vi "tt20panel_register_events.vi"(8 "error in (no error)":errorcluster, 11 "tt20panel in":refnum<class "tt20panel.lvclass">) -> (0 "error out":errorcluster, 2 "event_refs":T1, 3 "tt20panel out":refnum<class "tt20panel.lvclass">)   [LabVIEW 2015, in "tt20panel.lvclass"]
uses:
  tt20panel.lvclass
  tt20_evebnt_refs_tdef.ctl
  tt20_class/tt20_hardware_info_tdef.ctl
  tt20_acq_mode_tdef.ctl
  tt20_event_tdef.ctl
  tt20panel.lvclass/tt20panel.ctl
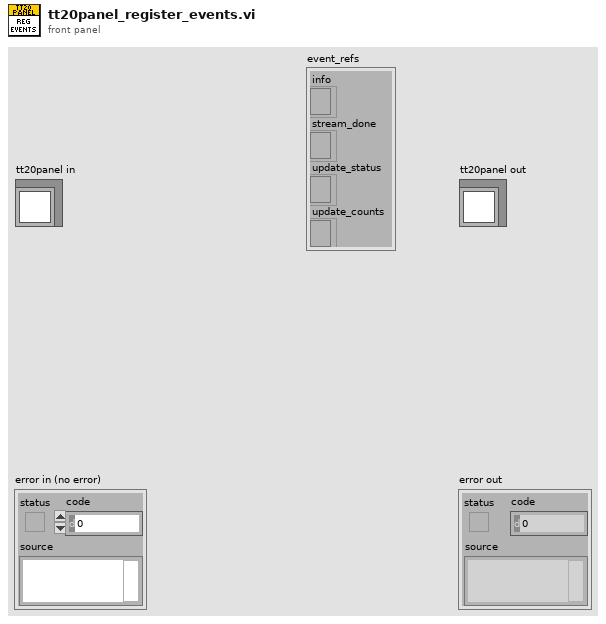
[diagram p1: front panel]
types:
  T1 = typedef "tt20_evebnt_refs_tdef.ctl" = cluster{"info":refnum<event-registration>, "stream_done":refnum<event-registration>, "update_status":refnum<event-registration>, "update_counts":refnum<event-registration>}
  T2 = typedef "tt20_event_tdef.ctl" = cluster{"tt20_get_info":refnum<user-event>, "stream_done":refnum<user-event>, "update_status":refnum<user-event>, "update_counts":refnum<user-event>}
  T3 = typedef "tt20_hardware_info_tdef.ctl" = cluster{"model":string, "serial":string, "trigger_level":dbl[], "input_delay":i64[], "deadtime":i64[], "num_channels":u32, "status":string, "enabled":bool[], "Mode":T4, "Reference Channel":u8}
  T4 = typedef "tt20_acq_mode_tdef.ctl" = enum16{"T2", "T3"}
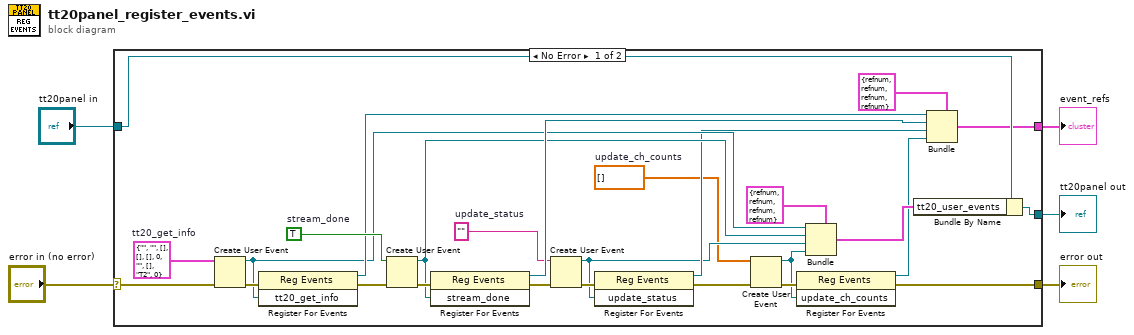
[diagram p0: block diagram]
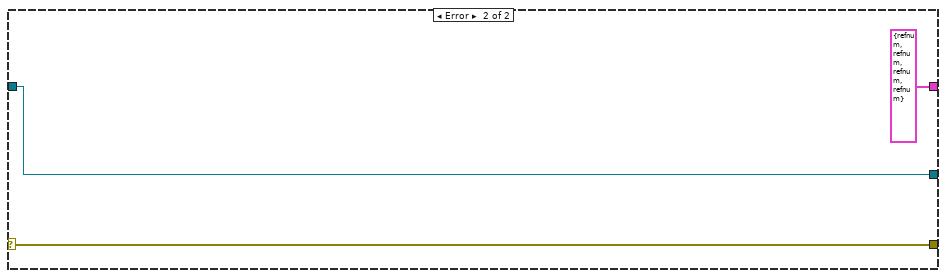
[diagram p2: hidden frame]
diagram:
  n1 = case shown="No Error" "error in (no error)" {
    selector: "error in (no error)" -> [w30 w35]
    tunnel: [w8 w35] -> w4
    tunnel: [w18 w34] -> w2
    tunnel: "tt20panel in" -> [w19 w34]
    tunnel: [w17 T1 {"info"=refnum, "stream_done"=refnum, "update_status"=refnum, "update_counts"=refnum} ("output cluster")] -> w1
    frame No Error {
      w10 = dbl[] []  # update_ch_counts
      w15 = ""  # update_status
      w31 = TRUE  # stream_done
      w32 = T3 {"model"="", "serial"="", "trigger_level"=[], "input_delay"=[], "deadtime"=[], "num_channels"=0, "status"="", "enabled"=[], "Mode"=enum."T2", "Reference Channel"=0}  # tt20_get_info
      n2 = Create User Event(user event datatype=w32, error in=w30) -> (user event=w23:refnum<user-event>, error out=w29:errorcluster)
      n3 = register-events(error in=w29, w23) -> (reference out=w25:refnum<event-registration>, error out=w28:errorcluster)  [unwired: 1 in]
      n4 = Create User Event(user event datatype=w31, error in=w28) -> (user event=w22:refnum<user-event>, error out=w27:errorcluster)
      n5 = register-events(error in=w27, w22) -> (reference out=w26:refnum<event-registration>, error out=w16:errorcluster)  [unwired: 1 in]
      n6 = Create User Event(user event datatype=w15, error in=w16) -> (user event=w12:refnum<user-event>, error out=w14:errorcluster)
      n7 = register-events(error in=w14, w12) -> (reference out=w13:refnum<event-registration>, error out=w11:errorcluster)  [unwired: 1 in]
      n8 = Create User Event(user event datatype=w10, error in=w11) -> (user event=w7:refnum<user-event>, error out=w9:errorcluster)
      n9 = register-events(error in=w9, w7) -> (reference out=w6:refnum<event-registration>, error out=w8:errorcluster)  [unwired: 1 in]
      n10 = Bundle(cluster=T2 {"tt20_get_info"=refnum, "stream_done"=refnum, "update_status"=refnum, "update_counts"=refnum} ("output cluster"), "tt20_get_info"=w23, "stream_done"=w22, "update_status"=w12, "update_counts"=w7) -> (w20:T2)
      n11 = Bundle By Name(cluster=w19, "tt20_user_events"=w20) -> (w18:refnum<class "tt20panel.lvclass">)
      n12 = Bundle(cluster=T1 {"info"=refnum, "stream_done"=refnum, "update_status"=refnum, "update_counts"=refnum} ("output cluster"), "info"=w25, "stream_done"=w26, "update_status"=w13, "update_counts"=w6) -> (w17:T1)
    }
    frame Error {
    }
  }
  "error out" <- w4
  "tt20panel out" <- w2
  "event_refs" <- w1
